vi "ISMBUS_ClosePort.vi"(8 "Fehler (Eingang - kein Fehler)":errorcluster) -> (0 "Fehler (Ausgang)":errorcluster)   [LabVIEW 2016]
uses:
  ISMBUS32.DLL
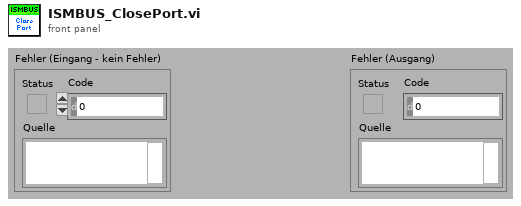
[diagram p1: front panel]
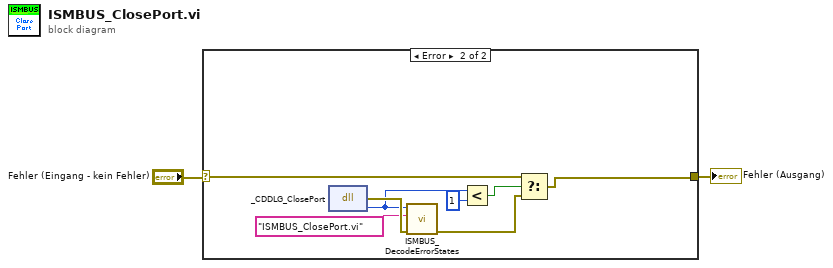
[diagram p0: block diagram]
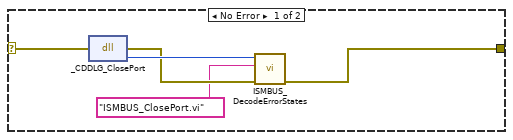
[diagram p2: hidden frame]
diagram:
  n1 = case shown="Error" "Fehler (Eingang - kein Fehler)" {
    selector: "Fehler (Eingang - kein Fehler)" -> [w7 w13]
    tunnel: [w3 w12] -> w1
    frame No Error {
      n2 = dll-call lib="ISMBUS32.DLL" fn="_CDDLG_ClosePort"(error in=w7) -> (error out=w5:errorcluster, "Rückgabetyp"=w6:i32)  [unwired: 2 in, 1 out]
      n3 = call "ISMBUS_DecodeErrorStates.vi"("Fehler (Eingang - kein Fehler)"=w5, "Location"="ISMBUS_ClosePort.vi", "ISMBUS_Error State"=w6) -> ("Fehler (Ausgang)"=w3:errorcluster)  [unwired: 8 in]
    }
    frame Error {
      n4 = dll-call lib="ISMBUS32.DLL" fn="_CDDLG_ClosePort"() -> (error out=w15:errorcluster, "Rückgabetyp"=w9:i32)  [unwired: 3 in, 1 out]
      n5 = call "ISMBUS_DecodeErrorStates.vi"("Fehler (Eingang - kein Fehler)"=w15, "Location"="ISMBUS_ClosePort.vi", "ISMBUS_Error State"=w9) -> ("Fehler (Ausgang)"=w11:errorcluster)  [unwired: 8 in]
      n6 = Less?(x=w9, y=1) -> (x < y?=w10:bool)
      n7 = Select(t=w13, s=w10, f=w11) -> (s? t:f=w12:errorcluster)
    }
  }
  "Fehler (Ausgang)" <- w1
